vi "Global 6.vi"() -> ()   [LabVIEW 2015]
panel:
  in  "GyroPlaceHolder":dbl
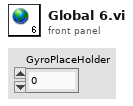
[diagram p1: front panel]
diagram:
